vi "test.vi"() -> ()   [LabVIEW 2012]
uses:
  TV/RW/Includes/WLAN - TV - OPPO - RW - INC - TV_Rx_Measurements.ctl
  TV/RW/Includes/WLAN - NIStandardDefine.ctl
panel:
  out "error out":errorcluster
  in  "Rx Measurements Settings":T1={"Channel Bandwidth (Hz)"=0.0, "Idle Interval (s)"=0.0, "80211n PLCP Frame Format"=0, "Payload Data Length (bytes)"=0, "OFDM Data Rate (Mbps)"=0, "DSSS Data Rate (Mbps)"=0, "#N_SS"=0, "NIStandard"=enum."80211B/G(DSSS)", "MCS Index"=""} {"DSSS Data Rate (Mbps)" items=["1", "2", "5.5 CCK", "5.5 PBCC", "11 CCK", "11 PBCC", "22", "33"]; "OFDM Data Rate (Mbps)" items=["6", "9", "12", "18", "24", "36", "48", "54"]; "80211n PLCP Frame Format" items=["Mixed Format", "Greenfield Format"]}
  in  "RFSG Handle":string
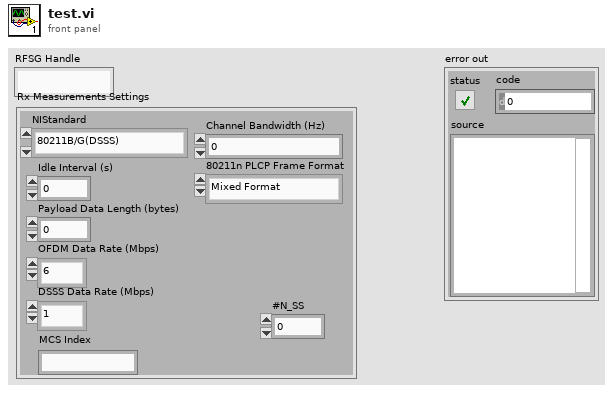
[diagram p1: front panel]
types:
  T1 = typedef "WLAN - TV - OPPO - RW - INC - TV_Rx_Measurements.ctl" = cluster{"Channel Bandwidth (Hz)":dbl, "Idle Interval (s)":dbl, "80211n PLCP Frame Format":i32, "Payload Data Length (bytes)":i32, "OFDM Data Rate (Mbps)":i32, "DSSS Data Rate (Mbps)":i32, "#N_SS":i32, "NIStandard":T2, "MCS Index":string}
  T2 = typedef "WLAN - NIStandardDefine.ctl" = enum32{"80211A/G/J/P(OFDM)", "80211B/G(DSSS)", "80211GDSSSOFDM", "80211NMIMOOFDM", "80211ACMIMOOFDM"}
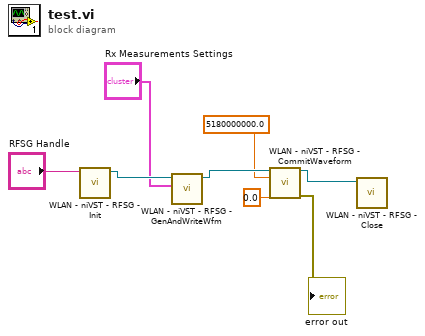
[diagram p0: block diagram]
diagram:
  n1 = call "WLAN - niVST - RFSG - Init.vi"("RFSG Handle"="RFSG Handle") -> ("RFSG handle out"=w7:refnum<k15>)  [unwired: 9 in, 1 out]
  n2 = call "WLAN - niVST - RFSG - GenAndWriteWfm.vi"("Rx Measurements Settings"="Rx Measurements Settings", "instrument handle"=w7) -> ("RFSG out"=w6:refnum<k15>)  [unwired: 8 in, 1 out]
  n3 = call "WLAN - niVST - RFSG - CommitWaveform.vi"("RFSG handle"=w6, "RF:Frequency (Hz)"=5180000000.0, "RxPower"=0.0) -> ("RFSG handle out"=w5:refnum<k15>, "error out"=→"error out":errorcluster)  [unwired: 11 in]
  n4 = call "WLAN - niVST - RFSG - Close.vi"("RFSG handle"=w5) -> ()  [unwired: 10 in, 1 out]
